vi "axis_GetPixelInfo.vi"(0 "Pixel Format":T1(ring)) -> (1 "Type":enum16{"JPG"}(ring), 2 "Width":u32, 3 "Height":u32)   [LabVIEW 2009]
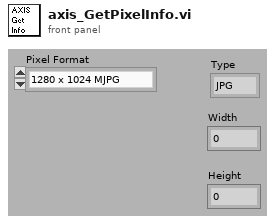
[diagram p1: front panel]
types:
  T1 = enum16{"1280 x 1024 MJPG", "1280 x 960 MJPG", "1280 x 720 MJPG", "1280 x 480 MJPG", "640 x 480 MJPG", "320 x 240 MJPG", "160 x 120 MJPG"}
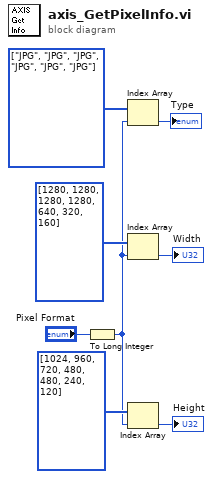
[diagram p0: block diagram]
diagram:
  w3 = enum16{"JPG"}[] [enum."JPG", enum."JPG", enum."JPG", enum."JPG", enum."JPG", enum."JPG"] items=["JPG"]
  n1 = To Long Integer(number="Pixel Format") -> (32bit integer=w2:i32)
  n2 = Index Array(array=w3, index=w2) -> (element=→"Type":enum16{"JPG"})
  n3 = Index Array(array=u32[] [1280, 1280, 1280, 1280, 640, 320, 160], index=w2) -> (element=→"Width":u32)
  n4 = Index Array(array=u32[] [1024, 960, 720, 480, 480, 240, 120], index=w2) -> (element=→"Height":u32)
